vi "Detect (Greyscale).vi"(5 "Non-Maxium Suppression Threshold":sgl, 7 "Confidence Threshold":sgl=0.5, 8 "error in (no error)":errorcluster, 10 "ARGB Image in":T4, 11 "DNN Detection Model in":refnum<class "DNN Detection Model.lvclass">) -> (0 "error out":errorcluster, 2 "Detections":T1[](array[typedef]), 3 "DNN Detection Model":refnum<class "DNN Detection Model.lvclass">)   [LabVIEW 2020, in "feature_detection.lvlib" / "DNN Detection Model.lvclass"]
uses:
  DNN Detection Model.lvclass
  image/Greyscale Image.ctl
  Detection.ctl
  Rectangle Corners.ctl
  common/Image Point (Integer).ctl
  DNN Detection Model.lvclass/DNN Detection Model.ctl
  e837249a-f575-44a9-ab73-66ed6d7d79a4.vi
  <vilib>/Utility/error.llb/Error Cluster From Error Code.vi
  image/image.lvlib
  common/common.lvlib
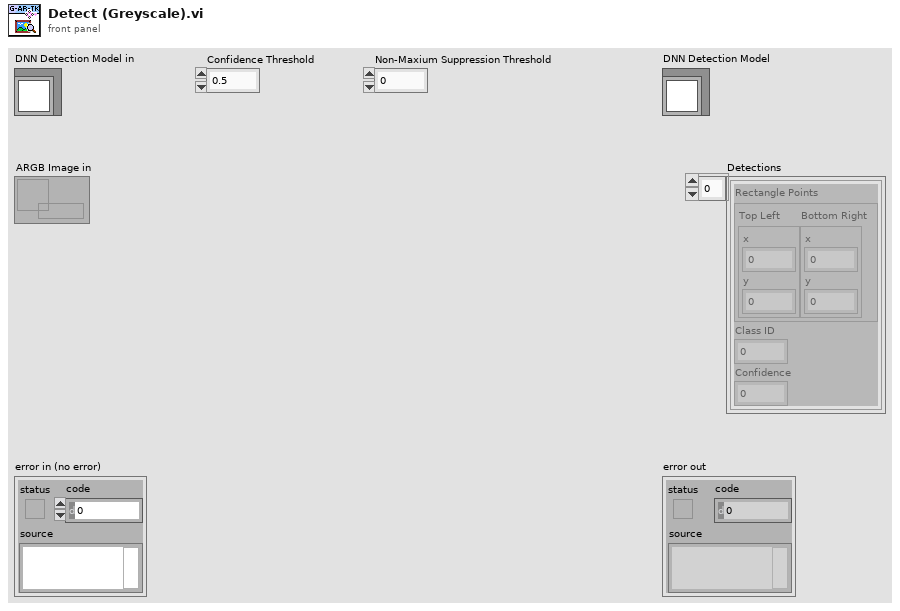
[diagram p1: front panel]
types:
  T1 = typedef "feature_detection.lvlib/DNN Detection Model.lvclass/Detection.ctl" = cluster{"Rectangle Points":T2, "Class ID":i32, "Confidence":sgl}
  T2 = typedef "feature_detection.lvlib/DNN Detection Model.lvclass/Rectangle Corners.ctl" = cluster{"Top Left":T3, "Bottom Right":T3}
  T3 = typedef "common.lvlib/Image Point (Integer).ctl" = cluster{"x":i32, "y":i32}
  T4 = typedef "image.lvlib/Greyscale Image.ctl" = refnum<data-value>
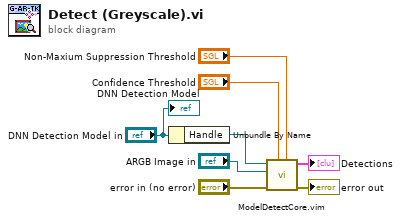
[diagram p0: block diagram]
diagram:
  n1 = Unbundle By Name("DNN Detection Model in") -> ("Handle"=w7:refnum<data-value>)
  n2 = call "ModelDetectCore.vim"("Non-Maxium Suppression Threshold"="Non-Maxium Suppression Threshold", "Confidence Threshold"="Confidence Threshold", "error in (no error)"="error in (no error)", "Image in"="ARGB Image in", "Detection Model"=w7) -> ("error out"=→"error out":errorcluster, "Detections"=→"Detections":T1[])  [unwired: 5 in]
  "DNN Detection Model" <- "DNN Detection Model in"
